vi "SetFlashValveState.vi"(7 "Timeout (ms)":u32=2000, 8 "Error In":errorcluster, 10 "Valve State":T1, 11 "Sierra M100 In":refnum<visa-resource-name>) -> (0 "Error Out":errorcluster, 2 "Set?":bool, 3 "Sierra M100 Out":refnum<visa-resource-name>)   [LabVIEW 2012, in "Sierra-M100.lvlib"]
doc: "This VI sets the state of the valve in Flash memory. Flash memory is non-volatile and the valve state will be retained during power cycling."
uses:
  Sierra-M100.lvlib
  Controls/ValveState.ctl
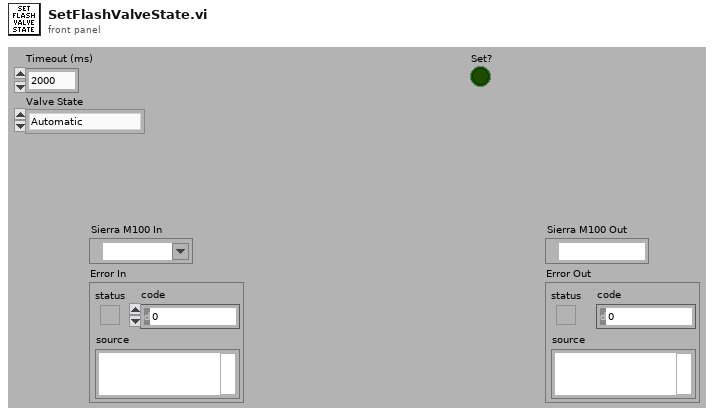
[diagram p1: front panel]
types:
  T1 = typedef "Sierra-M100.lvlib/ValveState.ctl" = enum16{"Automatic", "Closed", "Purge"}
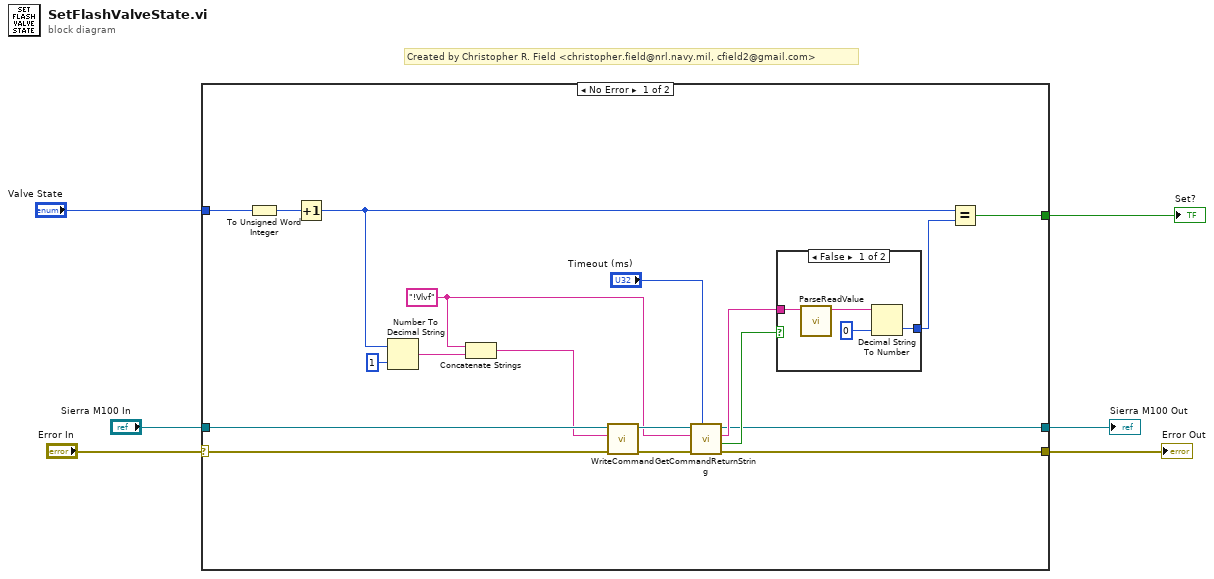
[diagram p0: block diagram]
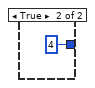
[diagram p2: hidden frame]
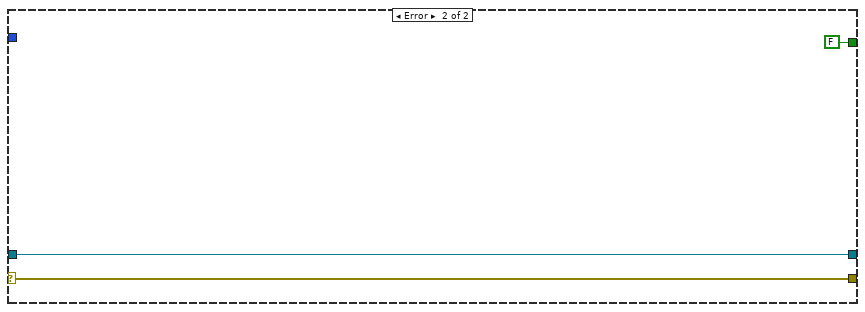
[diagram p3: hidden frame]
diagram:
  # "Created by Christopher R. Field <christopher.field@nrl.navy.mil, cfield2@gmail.com>"
  n1 = case shown="No Error" "Error In" {
    selector: "Error In" -> [w7 w31]
    tunnel: "Valve State" -> [w22 _]
    tunnel: "Sierra M100 In" -> [w20 w32]
    tunnel: [w12 w32] -> w5
    tunnel: [w11 w31] -> w4
    tunnel: [w8 FALSE] -> w3
    frame No Error {
      w16 = "!Vlvf"
      n2 = To Unsigned Word Integer(number=w22) -> (unsigned 16bit integer=w21:u16)
      n3 = Increment(x=w21) -> (x+1=w10:u16)
      n4 = Number To Decimal String(number=w10, width (-)=i16 1) -> (decimal integer string=w24:string)
      n5 = Concatenate Strings(w16, w24) -> (w19:string)
      n6 = call "WriteCommand.vi"("Error In"=w7, "Command"=w19, "Sierra M100 In"=w20) -> ("Error Out"=w17:errorcluster, "Sierra M100 Out"=w18:refnum<visa-resource-name>)  [unwired: 5 in, 2 out]
      n7 = call "GetCommandReturnString.vi"("Timeout (ms)"="Timeout (ms)", "Error In"=w17, "Command"=w16, "Sierra M100 In"=w18) -> ("Error Out"=w11:errorcluster, "Timeout?"=w13:bool, "Return String"=w14:string, "Sierra M100 Out"=w12:refnum<visa-resource-name>)  [unwired: 4 in]
      n8 = case shown="False" w13 {
        tunnel: w14 -> [w28 _]
        tunnel: [w25 u16 4] -> w9
        frame False {
          n9 = call "ParseReadValue.vi"("Read Buffer"=w28) -> ("Value"=w27:string)  [unwired: 10 in]
          n10 = Decimal String To Number(string=w27, default (0L)=u16 0 ("unsigned 16bit integer")) -> (number=w25:u16)  [unwired: 1 in, 1 out]
        }
        frame True {
        }
      }
      n11 = Equal?(x=w10, y=w9) -> (x = y?=w8:bool)
    }
    frame Error {
    }
  }
  "Sierra M100 Out" <- w5
  "Error Out" <- w4
  "Set?" <- w3
